vi "DIAdem Start.vi"(1 "error in (no error)":errorcluster, 2 "Data File (Path and File)":path) -> (0 "error out":errorcluster)   [LabVIEW 2020]
doc: "This VI calls DIAdem to generate a report containing graphs. A Wizard generates the report in DIAdem. Enter the name of the data file for which the report is to be generated as the VI \"Data File\" parameter. The LabVIEW ASCII spreadsheet file format is one of the data formats you can use. If you do not transfer a data file, a dialog for selecting data appears in the Wizard. \n\nDIAdem starts as an independent application. If one or more DIAdem applications are in use when you call the Report Wizard, the VI makes an OLE connection to the last one that was started."
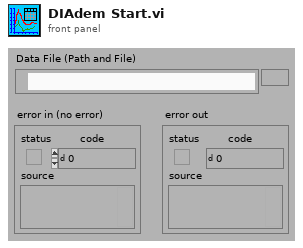
[diagram p1: front panel]
types:
  T1 = typedef "Window Refnum.ctl" = refnum<k1>
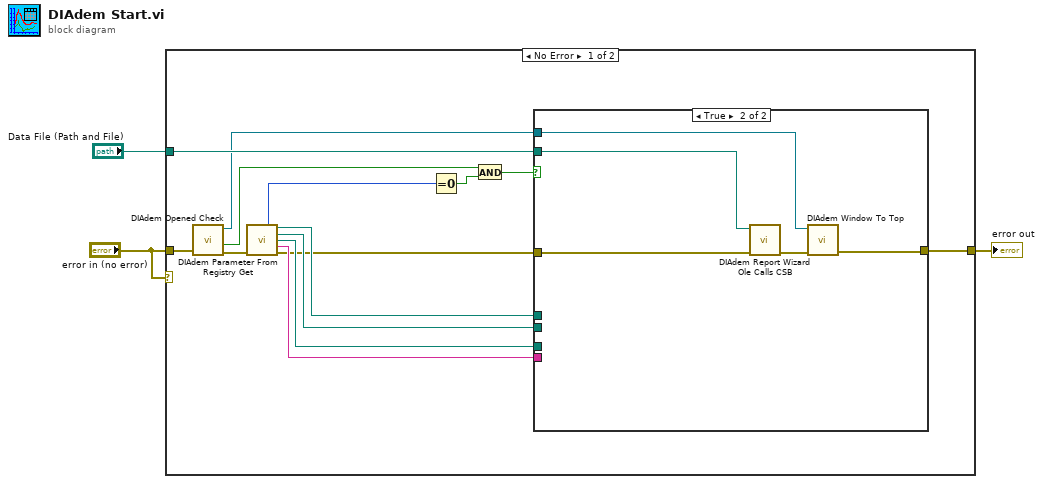
[diagram p0: block diagram]
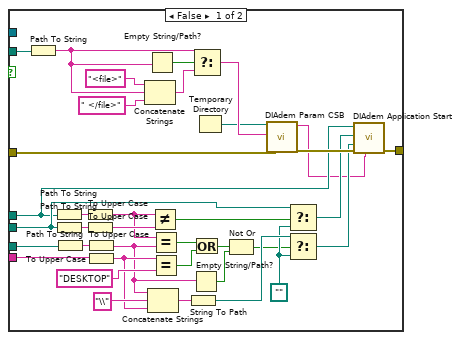
[diagram p2: hidden frame]
diagram:
  n1 = case shown="No Error" "error in (no error)" {
    tunnel: "Data File (Path and File)" -> [w13 _]
    tunnel: [w15 w59] -> w3
    tunnel: "error in (no error)" -> [w16 w59]
    frame No Error {
      n2 = call <vilib>:"DIAdem Opened Check.vi"("error in (no error)"=w16) -> ("DIAdem Window Refnum"=w11:T1, "DIAdem Opened"=w12:bool, "error out"=w10:errorcluster)  [unwired: 1 out]
      n3 = call <vilib>:"DIAdem Parameter From Registry Get.vi"("error in (no error)"=w10) -> ("DIAdem Application Directory"=w5:path, "DIAdem System Directory"=w8:path, "DIAdem Desktop Directory"=w7:path, "DIAdem Desktop File"=w6:string, "DIAdem Instancing Value"=w9:u32, "error out"=w4:errorcluster)  [unwired: 7 in, 2 out]
      n4 = Equal To 0?(x=w9) -> (x = 0?=w14:bool)
      n5 = And(x=w12, y=w14) -> (x .and. y?=w17:bool)
      n6 = case shown="True" w17 {
        tunnel: [w33 w56] -> w15
        tunnel: w13 -> [w27 w58]
        tunnel: w11 -> [_ w55]
        tunnel: w5 -> [w34 _]
        tunnel: w8 -> [w35 _]
        tunnel: w7 -> [w36 _]
        tunnel: w6 -> [w37 _]
        tunnel: w4 -> [w23 w54]
        frame False {
          w40 = path "" ("f")
          n7 = Path To String(path=w27) -> (string=w31:string)
          n8 = Path To String(path=w34) -> (string=w53:string)
          n9 = Path To String(path=w35) -> (string=w52:string)
          n10 = Path To String(path=w36) -> (string=w51:string)
          n11 = To Upper Case(1:w53) -> (0:w49:string)
          n12 = To Upper Case(1:w52) -> (0:w50:string)
          n13 = To Upper Case(1:w51) -> (0:w18:string)
          n14 = To Upper Case(1:w37) -> (0:w45:string)
          n15 = Concatenate Strings("<file>" ("Substring"), w31, " </file>" ("Substring")) -> (w28:string)
          n16 = Empty String/Path?(string/path=w31) -> (empty?=w32:bool)
          n17 = Concatenate Strings(w18, "\\" ("Substring"), w45) -> (w44:string)
          n18 = Not Equal?(x=w49, y=w50) -> (x != y?=w38:bool)
          n19 = Equal?(x=w49, y=w18) -> (x = y?=w41:bool)
          n20 = Equal?(x=w45, y="DESKTOP") -> (x = y?=w48:bool)
          n21 = String To Path(string=w44) -> (path=w43:path)
          n22 = Empty String/Path?(string/path=w18) -> (empty?=w20:bool)
          n23 = Select(t=w31, s=w32, f=w28) -> (s? t:f=w26:string)
          n24 = Or(x=w41, y=w48) -> (x .or. y?=w21:bool)
          n25 = Temporary Directory() -> (w22:path)
          n26 = Not Or(1:w20, 2:w21) -> (0:w19:bool)
          n27 = call <vilib>:"DIAdem Param CSB.vi"("error in (no error)"=w23, "Parameter"=w26, "File Directory"=w22) -> ("error out"=w42:errorcluster, "DIAdem Command Parameter"=w24:string)  [unwired: 3 in]
          n28 = Select(t=w35, s=w38, f=w40) -> (s? t:f=w39:path)
          n29 = Select(t=w43, s=w19, f=w40) -> (s? t:f=w25:path)
          n30 = call <vilib>:"DIAdem Application Start.vi"("DIAdem Additional Start Parameters"=w24, "error in (no error)"=w42, "DIAdem Desktop File"=w25, "DIAdem System Directory"=w39, "DIAdem Directory"=w34) -> ("error out"=w33:errorcluster)  [unwired: 4 in]
        }
        frame True {
          n31 = call <vilib>:"DIAdem Report Wizard Ole Calls CSB.vi"("error in (no error)"=w54, "Data File (Path and File)"=w58) -> ("error out"=w57:errorcluster)  [unwired: 9 in]
          n32 = call <vilib>:"DIAdem Window To Top.vi"("error in (no error)"=w57, "window refnum"=w55) -> ("error out"=w56:errorcluster)  [unwired: 5 in]
        }
      }
    }
    frame Error {
    }
  }
  "error out" <- w3
